vi "SeCrTs-PPSU Health.vi"(7 "Enum":enum16{"Read", "Write"}(ring), 8 "error in":errorcluster, 11 "ppsu health":bool) -> (0 "error out":errorcluster, 3 "ppsu health R":bool)   [LabVIEW 2022 SP3]
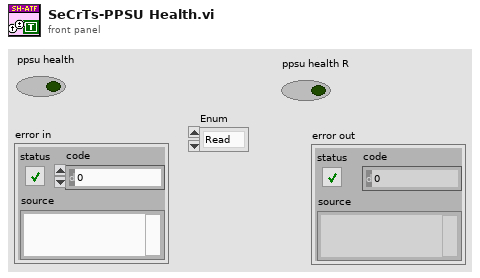
[diagram p1: front panel]
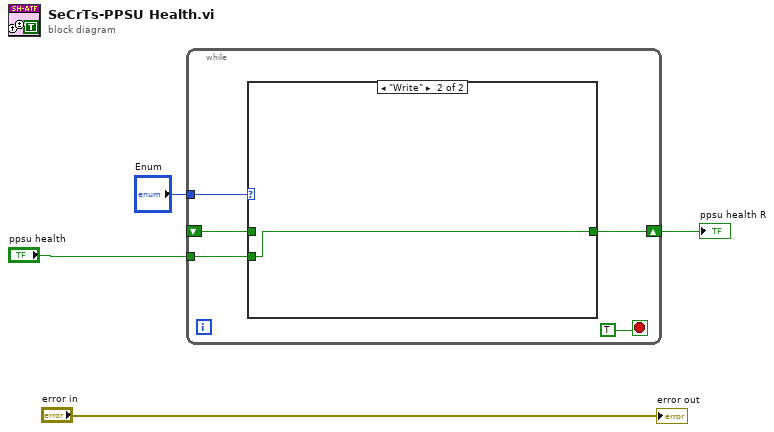
[diagram p0: block diagram]
diagram:
  n1 = while {
    tunnel: "Enum" -> [w9]
    tunnel: "ppsu health" -> [w7]
    shift-right: [w6] -> w1
    shift-left: _ -> [w5]
    stop <- TRUE stop-if-true
    n2 = case shown="\"Write\"" w9 {
      tunnel: w7 -> [_ w11]
      tunnel: [w10 w11] -> w6
      tunnel: w5 -> [w10 _]
      frame "Read", Default {
      }
      frame "Write" {
      }
    }
  }
  "ppsu health R" <- w1
  "error out" <- "error in"
